vi "FGV Read PV Protocols.vi"(8 "Error In":errorcluster, 9 "PVConnection in":refnum<class "PVConnection.lvclass">, 10 "PV Protocol":string) -> (0 "Error Out":errorcluster, 1 "PVConnection out":refnum<class "PVConnection.lvclass">, 2 "Success":bool, 4 "Protocols":string[](array[string]), 6 "PVConnections":refnum<class "PVConnection.lvclass">[](array[class]))   [LabVIEW 2015, in "CS++Base.lvlib"]
doc: "Read FGV maintaining a list of PV Connection protocolls."
uses:
  CS++Base.lvlib
  Classes/CS++ProcessVariables/PVConnection/PVConnection.lvclass
  FGV Action.ctl
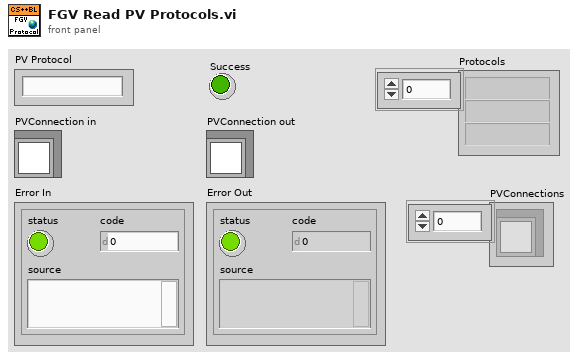
[diagram p1: front panel]
types:
  T1 = typedef "CS++Base.lvlib/FGV Action.ctl" = enum16{"add", "replace", "read", "remove", "reset", "get attributes"}
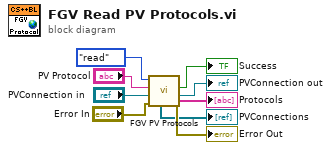
[diagram p0: block diagram]
diagram:
  n1 = call "FGV PV Protocols.vi"("Error In"="Error In", "PVConnection in"="PVConnection in", "PV Protocol"="PV Protocol", "Action (read)"=FGV_Action."read") -> ("Error Out"=→"Error Out":errorcluster, "PVConnection out"=→"PVConnection out":refnum<class "PVConnection.lvclass">, "Success"=→"Success":bool, "Protocols"=→"Protocols":string[], "PVConnections"=→"PVConnections":refnum<class "PVConnection.lvclass">[])  [unwired: 3 in]
